vi "PenaltyDefenseTactic.vi"(6 "PenaltyOurKick?":bool, 8 "error in (no error)":errorcluster, 9 "IndexInVector":dbl, 10 "Robot":refnum<class "Robot.lvclass">, 11 "PenaltyDefenseTactic in":refnum<class "PenaltyDefenseTactic.lvclass">) -> (0 "error out":errorcluster, 2 "Robot out":refnum<class "Robot.lvclass">, 3 "PenaltyDefenseTactic out":refnum<class "PenaltyDefenseTactic.lvclass">)   [LabVIEW 2018, in "PenaltyDefenseTactic.lvclass"]
uses:
  PenaltyDefenseTactic.lvclass
  C:/Users/yugon/Desktop/SSL_AI/SSL_AI/Tactic_class/Tactic.lvclass
  Robot_class/Robot.lvclass
  Tactic_class/Tactic.lvclass/Tactic.ctl
  Robot_class/tactics.ctl
  Skillbook_class/Skillbook.lvclass/Skillbook.ctl
  PenaltyDefenseTactic.lvclass/PenaltyDefenseTactic.ctl
  Robot_class/Robot.lvclass/Robot.ctl
  Skillbook_class/Read PenaltyDefenseSkill.vi
  Tactic_class/Read Skillbook.vi
  Robot_class/Write tactic.vi
  Write States.vi
  Skillbook_class/Skillbook.lvclass
  PenaltyDefenseSkill_class/PenaltyDefenseSkill.lvclass
panel:
  out "x .or. y?":bool
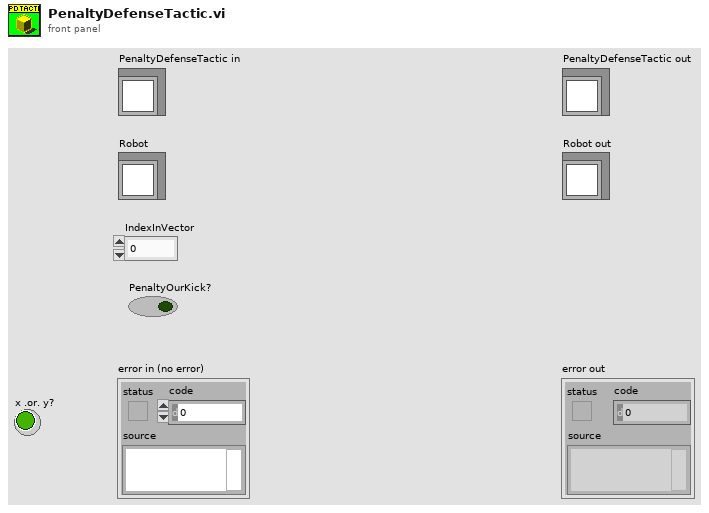
[diagram p1: front panel]
types:
  T1 = typedef "tactics.ctl" = enum16{"PenaltyAttacker", "PenaltyDefense", "Test", "DefendGoal", "Marker", "FollowAttacker", "DefendArea", "Shoot", "AttackerAimGoal", "AttackerBallOutOfField", "AttackerBlock", "AttackerStop", "Duelist", "Halt", "ZigZag", "GoTo", "Timeout", "KickToPassReceiver", "PositionToReceivePass", "PassReceiver", "WaitPass"}
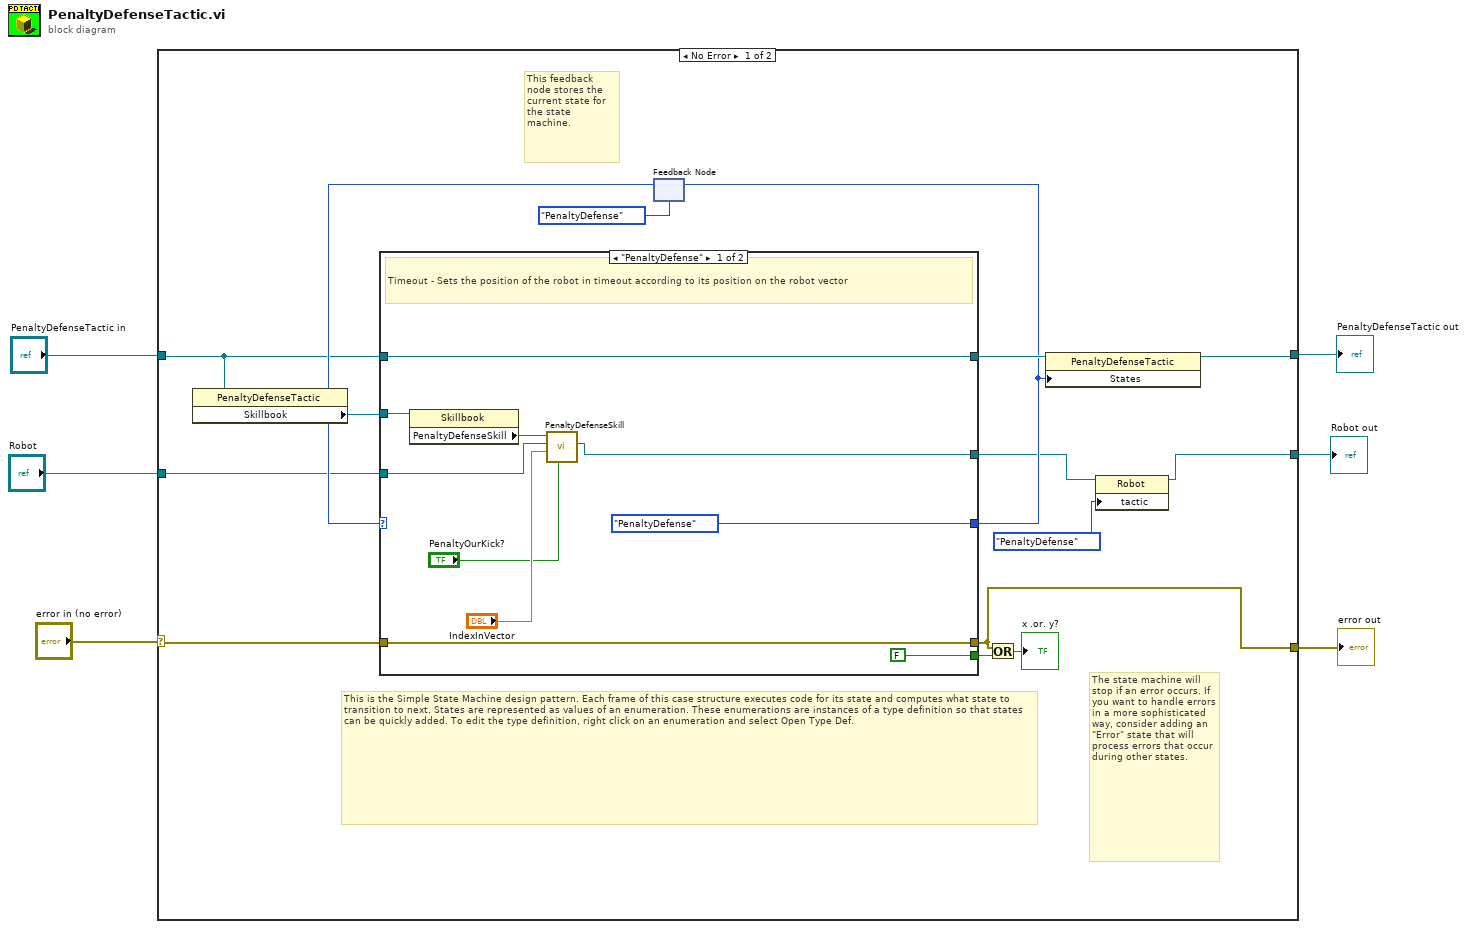
[diagram p0: block diagram]
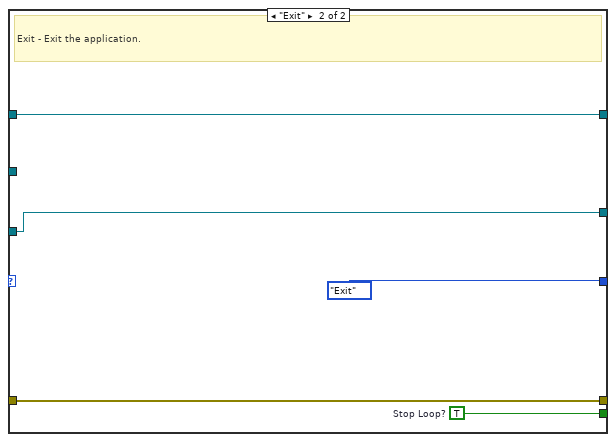
[diagram p2: hidden frame]
diagram:
  n1 = case shown="No Error" "error in (no error)" {
    selector: "error in (no error)" -> [w11 w39]
    tunnel: [w10 w39] -> w5
    tunnel: [w12 w38] -> w3
    tunnel: "PenaltyDefenseTactic in" -> [w14 w38]
    tunnel: "Robot" -> [w13 w37]
    tunnel: [w7 w37] -> w1
    frame No Error {
      # "The state machine will stop if an error occurs. If you want to handle errors in a more sophisticated way, consider adding an \"Error\" state that will process errors that occur during other states."
      # "This feedback node stores the current state for the state machine."
      # "This is the Simple State Machine design pattern. Each frame of this case structure executes code for its state and computes what state to transition to next. States are represented as values of an enumeration. These enumerations are instances of a type definition so that states can be quickly added. To edit the type definition, right click on an enumeration and select Open Type Def."
      n2 = property class="PenaltyDefenseTactic"(reference=w14) -> ("Skillbook"=w18:refnum<class "Skillbook.lvclass">)  [unwired: 1 in, 2 out]
      n3 = feedback #1(enum16{"Exit", "PenaltyDefense"}."PenaltyDefense" ("States")) -> (w19:enum16{"Exit", "PenaltyDefense"})
      n4 = case shown="\"PenaltyDefense\"" w19 {
        tunnel: [enum16{"Exit", "PenaltyDefense"}."PenaltyDefense" ("States") enum16{"Exit", "PenaltyDefense"}."Exit" ("States")] -> w16
        tunnel: [FALSE ("Stop Loop?") w36] -> w21
        tunnel: w18 -> [w30 _]
        tunnel: [w28 w33] -> w8
        tunnel: [w29 w35] -> w17
        tunnel: w14 -> [w29 w35]
        tunnel: w13 -> [w24 w33]
        tunnel: [w22 w32] -> w10
        tunnel: w11 -> [w22 w32]
        frame "PenaltyDefense" {
          # "Timeout - Sets the position of the robot in timeout according to its position on the robot vector"
          n5 = property class="Skillbook"(reference=w30) -> ("PenaltyDefenseSkill"=w25:refnum<class "PenaltyDefenseSkill.lvclass">)  [unwired: 1 in, 2 out]
          n6 = call-dynamic "PenaltyDefenseSkill.vi"("PenaltyOurKick?"="PenaltyOurKick?", "IndexInVector"="IndexInVector", "Robot"=w24, "PenaltyDefenseSkill in"=w25) -> ("Robot out"=w28:refnum<class "Robot.lvclass">)  [unwired: 5 in, 2 out]
        }
        frame "Exit" {
          w36 = TRUE  # Stop Loop?
          # "Exit - Exit the application."
        }
      }
      n7 = feedback-in #1(w16) -> ()
      n8 = Or(x=w10, y=w21) -> (x .or. y?=→"x .or. y?":bool)
      n9 = property class="PenaltyDefenseTactic"(reference=w17, "States"=w16) -> (reference out=w12:refnum<class "PenaltyDefenseTactic.lvclass">)  [unwired: 1 in, 1 out]
      n10 = property class="Robot"(reference=w8, "tactic"=tactics."PenaltyDefense") -> (reference out=w7:refnum<class "Robot.lvclass">)  [unwired: 1 in, 1 out]
    }
    frame Error {
    }
  }
  "error out" <- w5
  "PenaltyDefenseTactic out" <- w3
  "Robot out" <- w1
